vi "Transceiver Transmit.vi"(8 "error in (no error)":errorcluster, 10 "Transfer Group in":refnum<class "Transfer Group.lvclass">, 11 "Transceiver Thread in":refnum<class "Transceiver Thread.lvclass">) -> (0 "error out":errorcluster, 2 "Transfer Group out":refnum<class "Transfer Group.lvclass">, 3 "Transceiver Thread out":refnum<class "Transceiver Thread.lvclass">)   [LabVIEW 2019, in "DSF Core.lvlib" / "Transceiver Thread.lvclass"]
uses:
  Transceiver Thread.lvclass
  Transfer Group/Transfer Group.lvclass
  Transceiver Thread.lvclass/Transceiver Thread.ctl
  Transceiver/Transceiver.lvclass
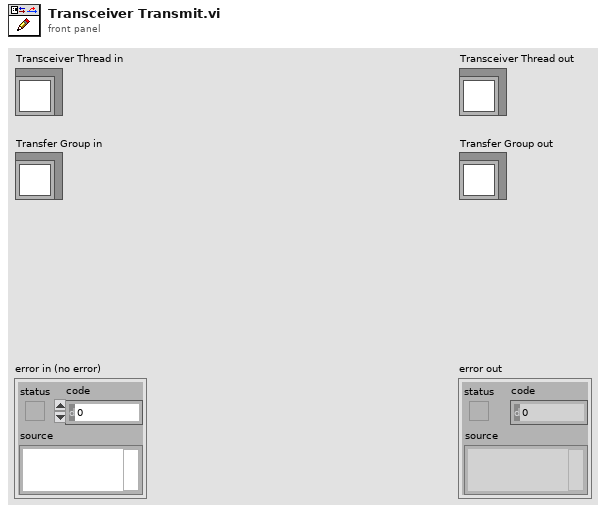
[diagram p1: front panel]
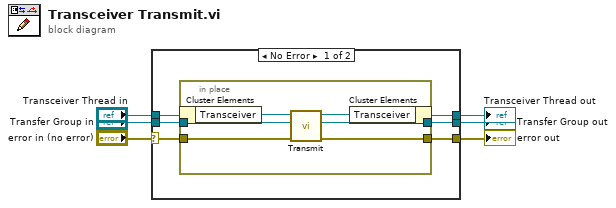
[diagram p0: block diagram]
diagram:
  n1 = case shown="No Error" "error in (no error)" {
    selector: "error in (no error)" -> [w7 w19]
    tunnel: "Transceiver Thread in" -> [w12 w21]
    tunnel: "Transfer Group in" -> [w11 w20]
    tunnel: [w10 w19] -> w4
    tunnel: [w9 w20] -> w3
    tunnel: [w8 w21] -> w2
    frame No Error {
      n2 = in-place {
        in-place-border: w7 -> [w18]
        in-place-border: w11 -> [w17]
        in-place-border: [w16] -> w10
        in-place-border: [w15] -> w9
        n3 = in-place-cluster #1(w12) -> ("Transceiver"=w14:refnum<class "Transceiver.lvclass">)
        n4 = call-dynamic "Transmit.vi"("error in (no error)"=w18, "Transfer Group in"=w17, "Transceiver in"=w14) -> ("error out"=w16:errorcluster, "Transfer Group out"=w15:refnum<class "Transfer Group.lvclass">, "Transceiver out"=w13:refnum<class "Transceiver.lvclass">)  [unwired: 6 in]
        n5 = in-place-cluster #1("Transceiver"=w13) -> (w8:refnum<class "Transceiver Thread.lvclass">)
      }
    }
    frame Error {
    }
  }
  "error out" <- w4
  "Transceiver Thread out" <- w2
  "Transfer Group out" <- w3
